vi "filter to array.vi"(8 "error in (no error)":errorcluster, 11 "name or relative path":string="Settings\\cDAQ\\filtri.txt") -> (0 "error out":errorcluster, 3 "filter array":T1(array[cluster]))   [LabVIEW 2019]
uses:
  <vilib>/Utility/file.llb/Read Delimited Spreadsheet (DBL).vi
panel:
  out "Array":dbl[](array[numeric])
  out "all rows":dbl[][](array[numeric])
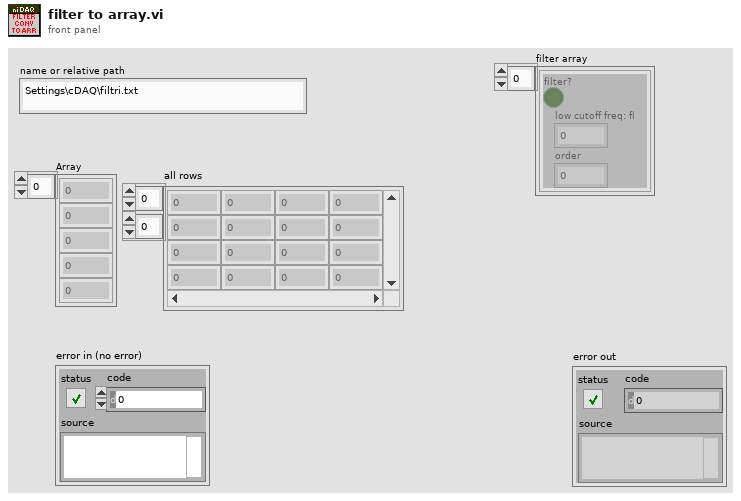
[diagram p1: front panel]
types:
  T1 = cluster{"filter?":bool, "low cutoff freq: fl":dbl, "order":i32}[]
  T2 = cluster{"filter?":bool, "low cutoff freq: fl":dbl, "order":i32}
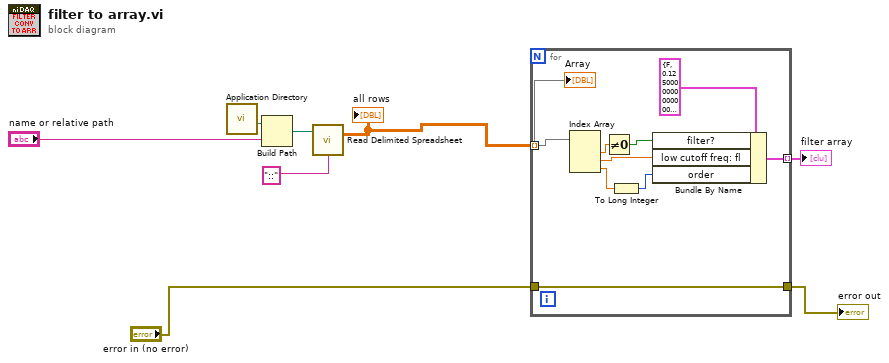
[diagram p0: block diagram]
diagram:
  n1 = call <vilib>:"Application Directory.vi"() -> ("Application Directory"=w8:path)
  n2 = Build Path(base path=w8, name or relative path="name or relative path") -> (appended path=w6:path)
  n3 = call-poly <vilib>:"Read Delimited Spreadsheet.vi"("file path (dialog if empty)"=w6, "delimiter (\\t)"="::" ("format (%.3f)")) -> ("all rows"=w4:dbl[][])  [unwired: 8 in, 5 out]
  "all rows" <- w4
  n4 = for {
    tunnel: w4 -> [w16] mode=indexing
    tunnel: [w10] -> w3 mode=indexing
    tunnel: "error in (no error)" -> [w9]
    tunnel: [w9] -> w1
    n5 = Index Array(array=w16) -> (element #1=w12:dbl, element #2=w15:dbl, element #3=w14:dbl)  [unwired: 3 in]
    n6 = Not Equal To 0?(x=w12) -> (x != 0?=w11:bool)
    n7 = To Long Integer(number=w14) -> (32bit integer=w13:i32)
    n8 = Bundle By Name(cluster=T2 {"filter?"=FALSE, "low cutoff freq: fl"=0.12500000000000006, "order"=2} ("Cluster"), "filter?"=w11, "low cutoff freq: fl"=w15, "order"=w13) -> (w10:T2)
    "Array" <- w16
  }
  "error out" <- w1
  "filter array" <- w3
